vi "Read Cursors Scroll Graph.vi"(8 "error in (no error)":errorcluster, 11 "IntensityGraph.lvclass in":refnum<class "IntensityGraph.lvclass">) -> (0 "error out":errorcluster, 2 "CrsrsScrollGrph":bool, 3 "IntensityGraph.lvclass out":refnum<class "IntensityGraph.lvclass">)   [LabVIEW 2015, in "IntensityGraph.lvclass"]
uses:
  IntensityGraph.lvclass
  IntensityGraph.lvclass/IntensityGraph.ctl
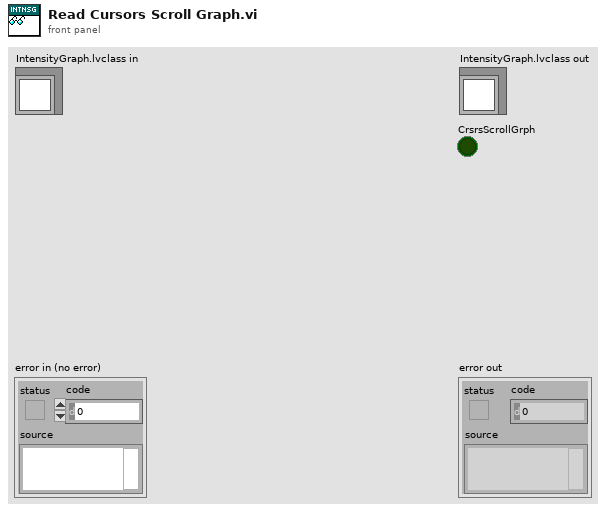
[diagram p1: front panel]
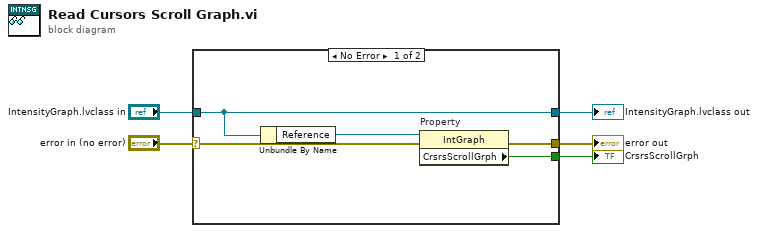
[diagram p0: block diagram]
diagram:
  n1 = case shown="No Error" "error in (no error)" {
    selector: "error in (no error)" -> [w6 w12]
    tunnel: [w9 w12] -> w4
    tunnel: [w8 w11] -> w2
    tunnel: "IntensityGraph.lvclass in" -> [w8 w11]
    tunnel: [w10 _] -> w1
    frame No Error {
      n2 = Unbundle By Name(w8) -> ("Reference"=w7:refnum<vi>)
      n3 = property on="Property" class="IntGraph"(reference=w7, error in=w6) -> (error out=w9:errorcluster, "CrsrsScrollGrph"=w10:bool)  [unwired: 1 out]
    }
    frame Error {
    }
  }
  "error out" <- w4
  "IntensityGraph.lvclass out" <- w2
  "CrsrsScrollGrph" <- w1
